vi "EmalBDD_pw.vi"(8 "Error in":errorcluster caption="Entrée d'erreur", 11 "PWattendu":u32=1234 caption="Mot de passe attendu") -> (0 "Error Out":errorcluster caption="Sortie d'erreur", 3 "pwOK?":bool)   [LabVIEW 2020]
panel:
  in  "btn_ok":bool
  in  "btn_index_c":bool
  in  "btn_index_0":bool
  in  "btn_index_9":bool
  in  "btn_index_8":bool
  in  "btn_index_7":bool
  in  "btn_index_6":bool
  in  "btn_index_5":bool
  in  "btn_index_4":bool
  in  "btn_index_3":bool
  in  "btn_index_2":bool
  in  "btn_index_1":bool
  in  "PW":u32 caption="Mot de passe \"maintenance\"" max=9999 format="%04.0f"
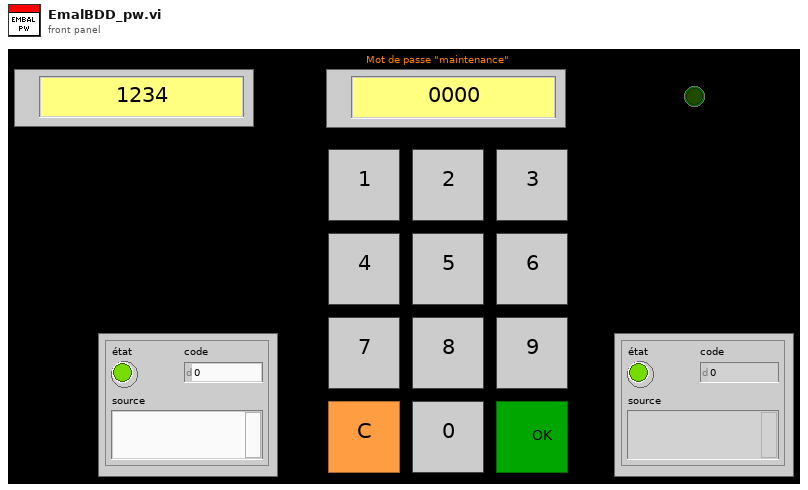
[diagram p1: front panel]
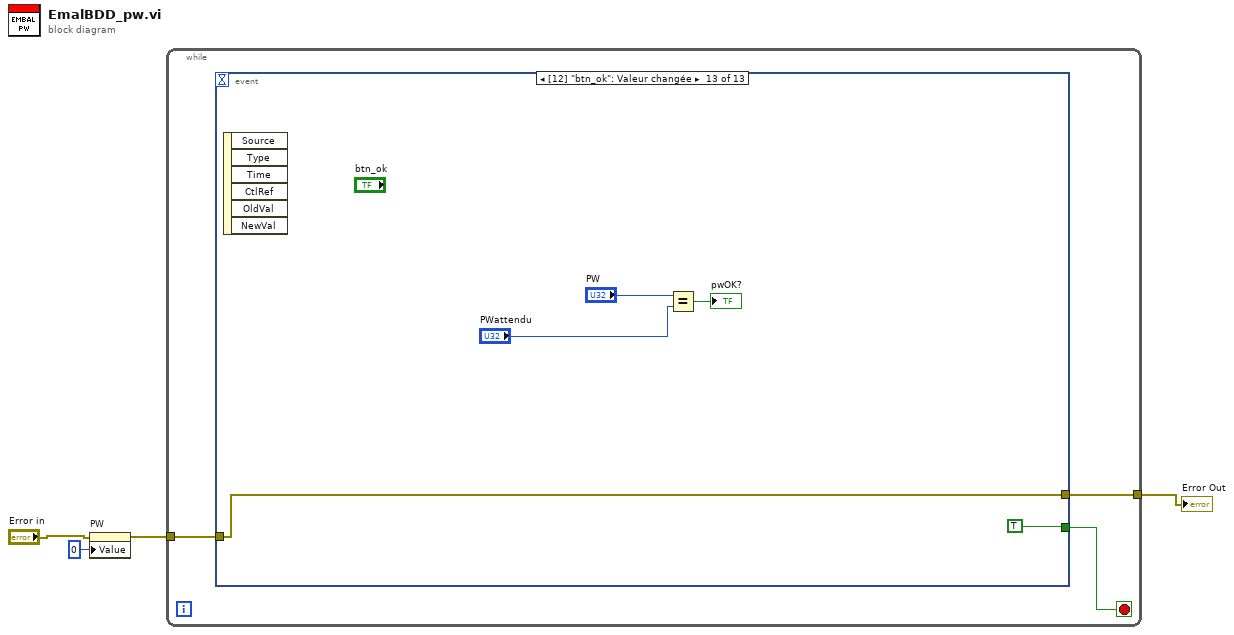
[diagram p0: block diagram]
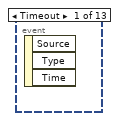
[diagram p2: hidden frame]
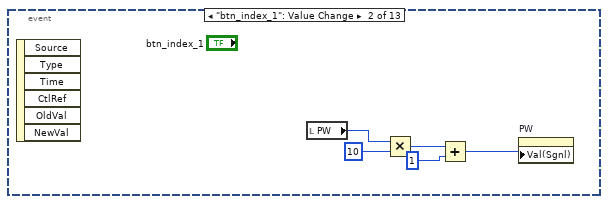
[diagram p3: hidden frame]
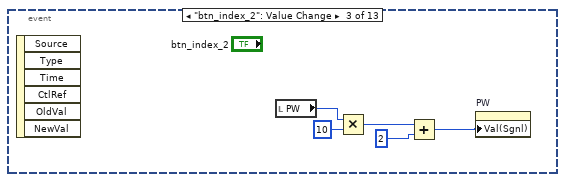
[diagram p4: hidden frame]
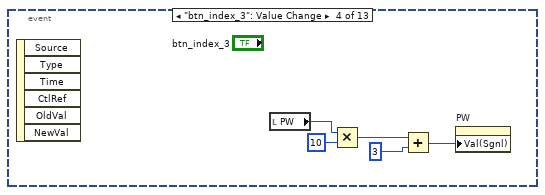
[diagram p5: hidden frame]
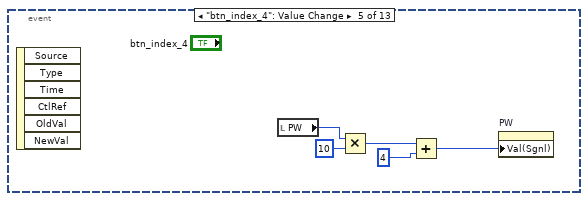
[diagram p6: hidden frame]
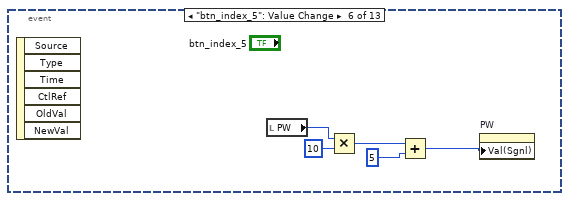
[diagram p7: hidden frame]
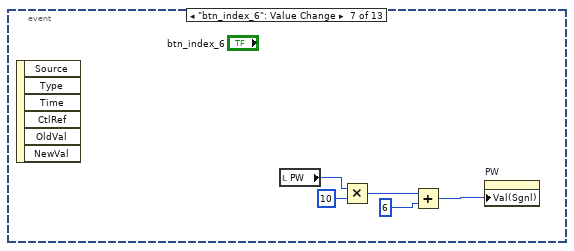
[diagram p8: hidden frame]
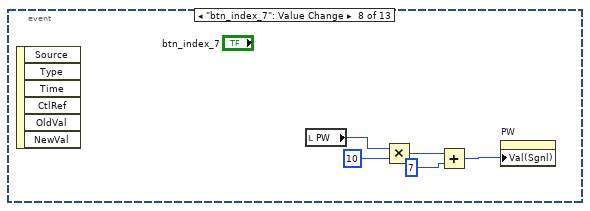
[diagram p9: hidden frame]
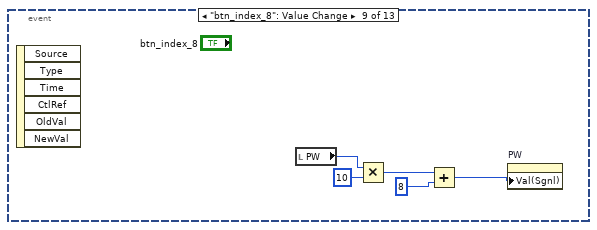
[diagram p10: hidden frame]
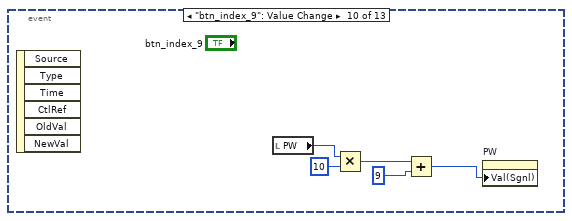
[diagram p11: hidden frame]
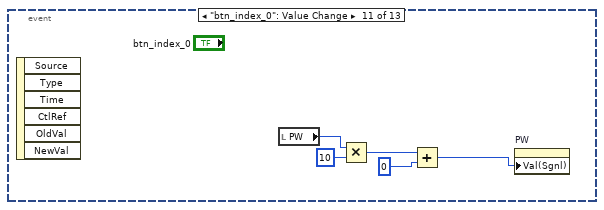
[diagram p12: hidden frame]
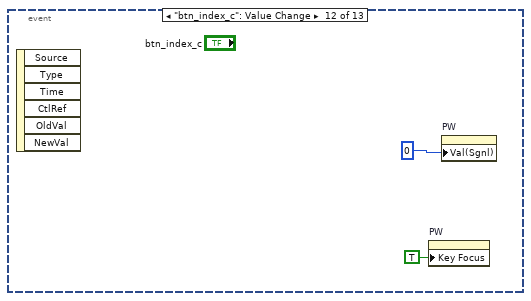
[diagram p13: hidden frame]
diagram:
  n1 = property on="PW" class="NumNb (strict)"(error in="Error in", "Value"=u32 0 ("PW")) -> (error out=w3:errorcluster)  [unwired: 1 in, 1 out]
  n2 = while {
    tunnel: w3 -> [w6]
    tunnel: [w5] -> w1
    stop <- w7 stop-if-true
    n3 = event shown="[12] \"btn_ok\": Valeur changée" {
      selector: _ -> [_ _ _ _ _ _ _ _ _ _ _ _ _]
      dyn-events: _ -> [_ _ _ _ _ _ _ _ _ _ _ _ _]
      timeout: _ -> [_ _ _ _ _ _ _ _ _ _ _ _ _]
      tunnel: [_ _ _ _ _ _ _ _ _ _ _ _ TRUE] -> w7
      tunnel: w6 -> [_ _ _ _ _ _ _ _ _ _ _ _ w60]
      tunnel: [_ _ _ _ _ _ _ _ _ _ _ _ w60] -> w5
      event Timeout {
        n4 = event-data() -> ()  [unwired: 1 in, 3 out]
      }
      event "btn_index_1": Value Change {
        n5 = event-data() -> ()  [unwired: 1 in, 6 out]
        n6 = local read "PW"() -> (w9:u32)
        n7 = Multiply(x=w9, y=u32 10) -> (x*y=w11:u32)
        n8 = Add(x=w11, y=u32 1) -> (x+y=w8:u32)
        n9 = property on="PW" class="NumNb (strict)"("Val(Sgnl)"=w8) -> ()  [unwired: 2 in, 2 out]
      }
      event "btn_index_2": Value Change {
        n10 = event-data() -> ()  [unwired: 1 in, 6 out]
        n11 = local read "PW"() -> (w14:u32)
        n12 = Multiply(x=w14, y=u32 10) -> (x*y=w16:u32)
        n13 = Add(x=w16, y=u32 2) -> (x+y=w13:u32)
        n14 = property on="PW" class="NumNb (strict)"("Val(Sgnl)"=w13) -> ()  [unwired: 2 in, 2 out]
      }
      event "btn_index_3": Value Change {
        n15 = event-data() -> ()  [unwired: 1 in, 6 out]
        n16 = local read "PW"() -> (w19:u32)
        n17 = Multiply(x=w19, y=u32 10) -> (x*y=w21:u32)
        n18 = Add(x=w21, y=u32 3) -> (x+y=w18:u32)
        n19 = property on="PW" class="NumNb (strict)"("Val(Sgnl)"=w18) -> ()  [unwired: 2 in, 2 out]
      }
      event "btn_index_4": Value Change {
        n20 = event-data() -> ()  [unwired: 1 in, 6 out]
        n21 = local read "PW"() -> (w24:u32)
        n22 = Multiply(x=w24, y=u32 10) -> (x*y=w26:u32)
        n23 = Add(x=w26, y=u32 4) -> (x+y=w23:u32)
        n24 = property on="PW" class="NumNb (strict)"("Val(Sgnl)"=w23) -> ()  [unwired: 2 in, 2 out]
      }
      event "btn_index_5": Value Change {
        n25 = event-data() -> ()  [unwired: 1 in, 6 out]
        n26 = local read "PW"() -> (w29:u32)
        n27 = Multiply(x=w29, y=u32 10) -> (x*y=w31:u32)
        n28 = Add(x=w31, y=u32 5) -> (x+y=w28:u32)
        n29 = property on="PW" class="NumNb (strict)"("Val(Sgnl)"=w28) -> ()  [unwired: 2 in, 2 out]
      }
      event "btn_index_6": Value Change {
        n30 = event-data() -> ()  [unwired: 1 in, 6 out]
        n31 = local read "PW"() -> (w34:u32)
        n32 = Multiply(x=w34, y=u32 10) -> (x*y=w36:u32)
        n33 = Add(x=w36, y=u32 6) -> (x+y=w33:u32)
        n34 = property on="PW" class="NumNb (strict)"("Val(Sgnl)"=w33) -> ()  [unwired: 2 in, 2 out]
      }
      event "btn_index_7": Value Change {
        n35 = event-data() -> ()  [unwired: 1 in, 6 out]
        n36 = local read "PW"() -> (w39:u32)
        n37 = Multiply(x=w39, y=u32 10) -> (x*y=w41:u32)
        n38 = Add(x=w41, y=u32 7) -> (x+y=w38:u32)
        n39 = property on="PW" class="NumNb (strict)"("Val(Sgnl)"=w38) -> ()  [unwired: 2 in, 2 out]
      }
      event "btn_index_8": Value Change {
        n40 = event-data() -> ()  [unwired: 1 in, 6 out]
        n41 = local read "PW"() -> (w44:u32)
        n42 = Multiply(x=w44, y=u32 10) -> (x*y=w46:u32)
        n43 = Add(x=w46, y=u32 8) -> (x+y=w43:u32)
        n44 = property on="PW" class="NumNb (strict)"("Val(Sgnl)"=w43) -> ()  [unwired: 2 in, 2 out]
      }
      event "btn_index_9": Value Change {
        n45 = event-data() -> ()  [unwired: 1 in, 6 out]
        n46 = local read "PW"() -> (w49:u32)
        n47 = Multiply(x=w49, y=u32 10) -> (x*y=w51:u32)
        n48 = Add(x=w51, y=u32 9) -> (x+y=w48:u32)
        n49 = property on="PW" class="NumNb (strict)"("Val(Sgnl)"=w48) -> ()  [unwired: 2 in, 2 out]
      }
      event "btn_index_0": Value Change {
        n50 = event-data() -> ()  [unwired: 1 in, 6 out]
        n51 = local read "PW"() -> (w54:u32)
        n52 = Multiply(x=w54, y=u32 10) -> (x*y=w56:u32)
        n53 = Add(x=w56, y=u32 0) -> (x+y=w53:u32)
        n54 = property on="PW" class="NumNb (strict)"("Val(Sgnl)"=w53) -> ()  [unwired: 2 in, 2 out]
      }
      event "btn_index_c": Value Change {
        n55 = event-data() -> ()  [unwired: 1 in, 6 out]
        n56 = property on="PW" class="NumNb (strict)"("Key Focus"=TRUE ("Focus clavier")) -> ()  [unwired: 2 in, 2 out]
        n57 = property on="PW" class="NumNb (strict)"("Val(Sgnl)"=u32 0 ("ID_Article")) -> ()  [unwired: 2 in, 2 out]
      }
      event "btn_ok": Value Change {
        n58 = event-data() -> ()  [unwired: 1 in, 6 out]
        n59 = Equal?(x="PW", y="PWattendu") -> (x = y?=→"pwOK?":bool)
      }
    }
  }
  "Error Out" <- w1
